vi "Empty.vi"(0 "object in":refnum<class "CetoniPump.lvclass">, 5 "error in (no error)":errorcluster) -> (14 "object out":refnum<class "CetoniPump.lvclass">, 19 "error out":errorcluster)   [LabVIEW 2024, in "CetoniPump.lvclass"]
uses:
  CetoniPump.lvclass
  CetoniPump.lvclass/CetoniPump.ctl
  Users/Lab user/AppData/Local/CETONI_SDK/lib/labview/labbCAN_Pump_API/labbCAN_Pump_API.lvlib
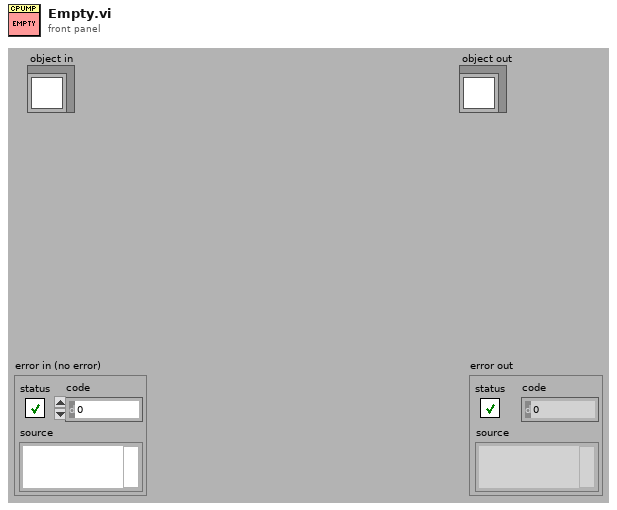
[diagram p1: front panel]
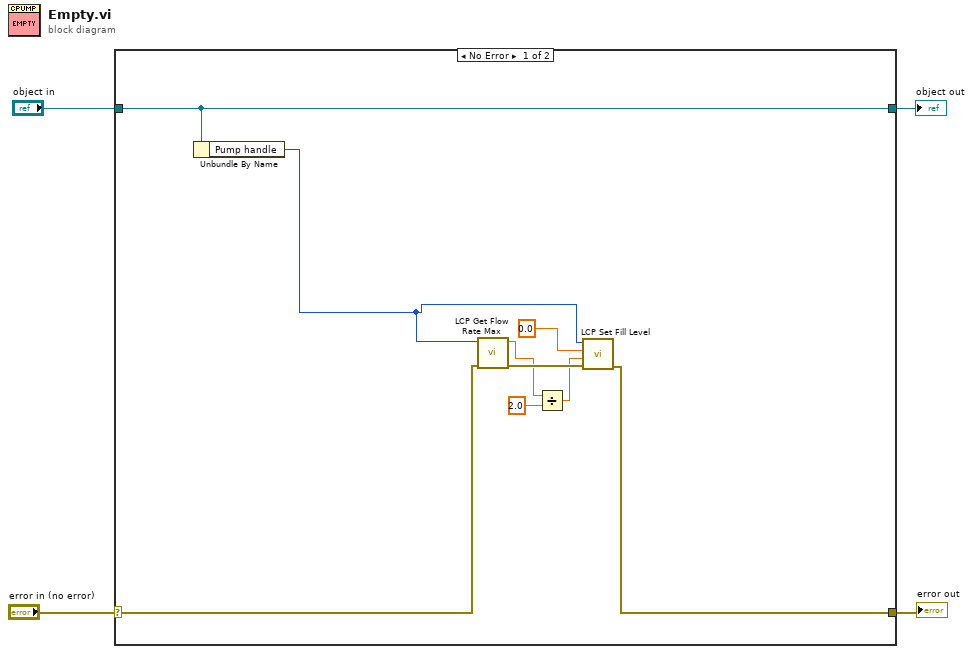
[diagram p0: block diagram]
diagram:
  n1 = case shown="No Error" "error in (no error)" {
    selector: "error in (no error)" -> [w9 w15]
    tunnel: [w8 w15] -> w3
    tunnel: [w13 w14] -> w1
    tunnel: "object in" -> [w13 w14]
    frame No Error {
      n2 = Unbundle By Name(w13) -> ("Pump handle"=w10:i64)
      n3 = call "LCP Get Flow Rate Max.vi"("error in (no error)"=w9, "Pump Handle"=w10) -> ("error out"=w12:errorcluster, "Maximum Flow Rate"=w7:dbl)  [unwired: 8 in]
      n4 = Divide(x=w7, y=2.0) -> (x/y=w6:dbl)
      n5 = call "LCP Set Fill Level.vi"("error in (no error)"=w12, "Flow"=w6, "Level"=0.0, "Pump Handle"=w10) -> ("error out"=w8:errorcluster)  [unwired: 7 in]
    }
    frame Error {
    }
  }
  "error out" <- w3
  "object out" <- w1
